vi "New Root Logger Normal.vi"(8 "error in (no error)":errorcluster) -> (0 "error out":errorcluster, 2 "logger normal":refnum<class "Logger Normal.lvclass">)   [LabVIEW 2020, in "Logger Normal.lvlib" / "Logger Normal.lvclass"]
uses:
  Logger Normal.lvclass
  <vilib>/ActorFramework/Actor/Actor.lvclass
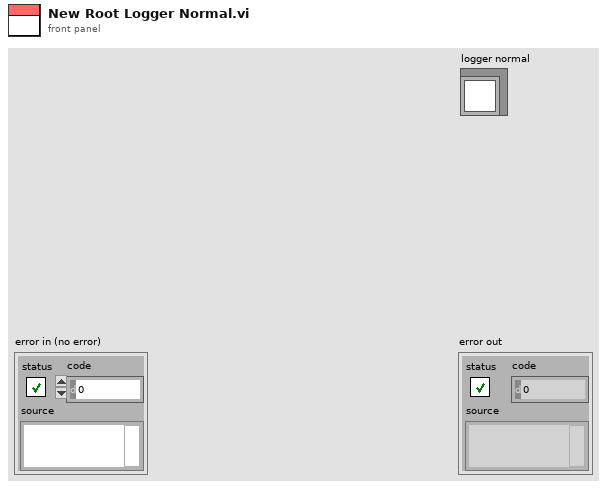
[diagram p1: front panel]
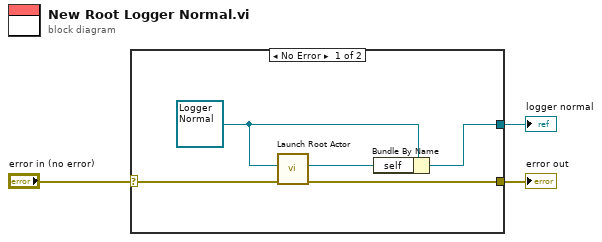
[diagram p0: block diagram]
diagram:
  n1 = case shown="No Error" "error in (no error)" {
    selector: "error in (no error)" -> [w8 w9]
    tunnel: [w5 w9] -> w2
    tunnel: [w4 _] -> w1
    frame No Error {
      w7 = refnum<class "Logger Normal.lvclass"> refnum ("Logger Normal in")
      n2 = call <vilib>:"Launch Root Actor.vi"("error in (no error)"=w8, "Actor"=w7) -> ("error out"=w5:errorcluster, "Actor's Enqueuer"=w6:refnum<class "Message Enqueuer.lvclass">)  [unwired: 8 in]
      n3 = Bundle By Name(cluster=w7, "self"=w6) -> (w4:refnum<class "Logger Normal.lvclass">)
    }
    frame Error {
    }
  }
  "error out" <- w2
  "logger normal" <- w1
